vi "Create.vi"(8 "error in (no error)":errorcluster, 9 "ID":i32, 10 "Name":string, 11 "Motor in":refnum<class "Motor-Xaxis.lvclass">) -> (0 "error out":errorcluster, 3 "Motor out":refnum<class "Motor-Xaxis.lvclass">)   [LabVIEW 2013, in "PowderDeposition.lvlib" / "Motor-Xaxis.lvclass"]
uses:
  Motor-Xaxis.lvclass
  Units.ctl
  Action-settings.ctl
  Motor.lvclass
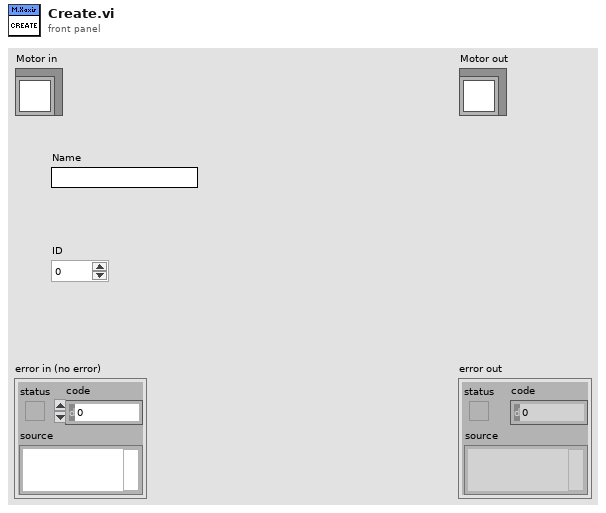
[diagram p1: front panel]
types:
  T1 = cluster{"deviceName":string, "protocolStackName":string, "interfaceName":string, "portName":string, "baudrate":u32, "timeout":u32}
  T2 = typedef "PowderDeposition.lvlib/Motor.lvclass/Action-settings.ctl" = cluster{"Speed":dbl, "Acceleration":dbl, "Direction":enum16{"Clockwise", "Counter-clockwise"}}
  T3 = typedef "PowderDeposition.lvlib/Motor.lvclass/Units.ctl" = enum16{"-", "mm", "µm", "tr", "V"}
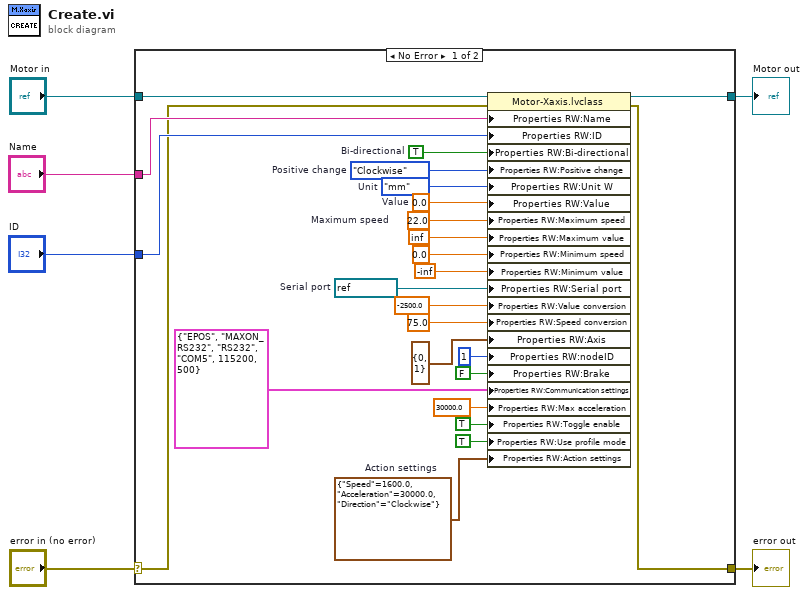
[diagram p0: block diagram]
diagram:
  n1 = case shown="No Error" "error in (no error)" {
    selector: "error in (no error)" -> [w7 w33]
    tunnel: [w8 w33] -> w5
    tunnel: [w9 w32] -> w3
    tunnel: "Motor in" -> [w31 w32]
    tunnel: "Name" -> [w30 _]
    tunnel: "ID" -> [w29 _]
    frame No Error {
      w17 = T2 {"Speed"=1600.0, "Acceleration"=30000.0, "Direction"=enum."Clockwise"}  # Action settings
      w20 = refnum<visa-resource-name> "COM5"  # Serial port
      w24 = 22.0  # Maximum speed
      w25 = 0.0  # Value
      w26 = Units."mm"  # Unit
      w27 = enum16{"Clockwise", "Counter-clockwise"}."Clockwise"  # Positive change
      w28 = TRUE  # Bi-directional
      n2 = property class="Motor-Xaxis.lvclass"(reference=w31, error in=w7, "Properties RW:Name"=w30, "Properties RW:ID"=w29, "Properties RW:Bi-directional"=w28, "Properties RW:Positive change"=w27, "Properties RW:Unit W"=w26, "Properties RW:Value"=w25, "Properties RW:Maximum speed"=w24, "Properties RW:Maximum value"=inf, "Properties RW:Minimum speed"=0.0 ("Minimum voltage"), "Properties RW:Minimum value"=-inf, "Properties RW:Serial port"=w20, "Properties RW:Value conversion"=-2500.0 ("Volt per tr/min."), "Properties RW:Speed conversion"=75.0 ("Volt conversion"), "Properties RW:Axis"=cluster{"keyHandle":u32, "nodeID":u16} {"keyHandle"=0, "nodeID"=1} ("Axis"), "Properties RW:nodeID"=u16 1 ("nodeID"), "Properties RW:Brake"=FALSE ("Brake"), "Properties RW:Communication settings"=T1 {"deviceName"="EPOS", "protocolStackName"="MAXON_RS232", "interfaceName"="RS232", "portName"="COM5", "baudrate"=115200, "timeout"=500} ("Communication settings"), "Properties RW:Max acceleration"=30000.0 ("Max acceleration"), "Properties RW:Toggle enable"=TRUE ("Toggle enable"), "Properties RW:Use profile mode"=TRUE ("Use profile mode"), "Properties RW:Action settings"=w17) -> (reference out=w9:refnum<class "Motor-Xaxis.lvclass">, error out=w8:errorcluster)
    }
    frame Error {
    }
  }
  "error out" <- w5
  "Motor out" <- w3
